vi "Select_Strings.vi"(4 "Timeout (s)":dbl=nan, 5 "Available Ch names":string[](array[string]), 6 "Message":string, 7 "Selector mode":T1(ring), 8 "Desired Ch names (in)":string[](array[string])) -> (0 "Ch Indicies Chosen":i32[](array[numeric]), 1 "Cancel":bool, 2 "Selected Channel Names":string[](array[string]))   [LabVIEW 2016]
panel:
  out "Auto-dismiss":dbl(slide) scale=0.0..60.0
  in  "Cancel 1":bool
  in  "OK":bool
  in  "Search String":string
  in  "Selector":i32[](listbox)
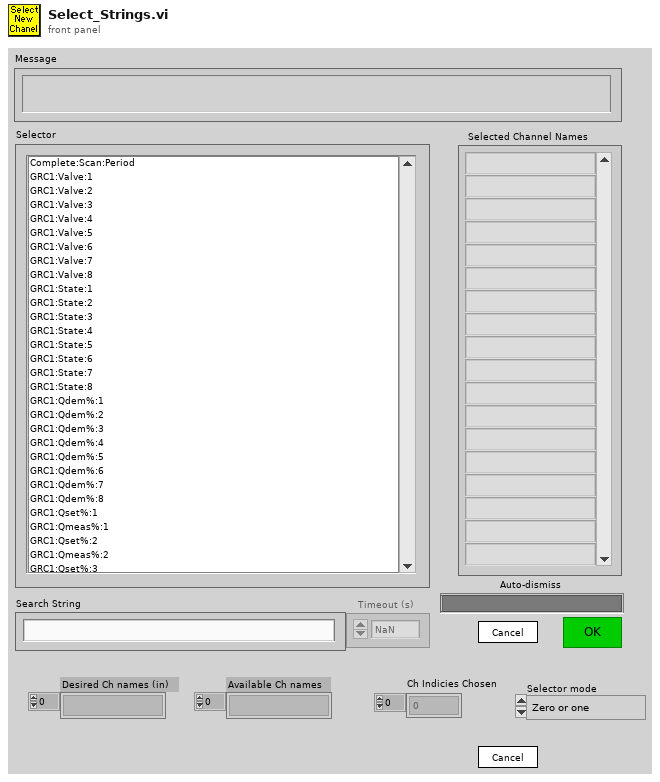
[diagram p1: front panel]
types:
  T1 = enum16{"Zero or one", "One", "Zero or more", "One or more"}
  T2 = enum8{"Enabled", "Disabled", "Disabled and Grayed Out"}
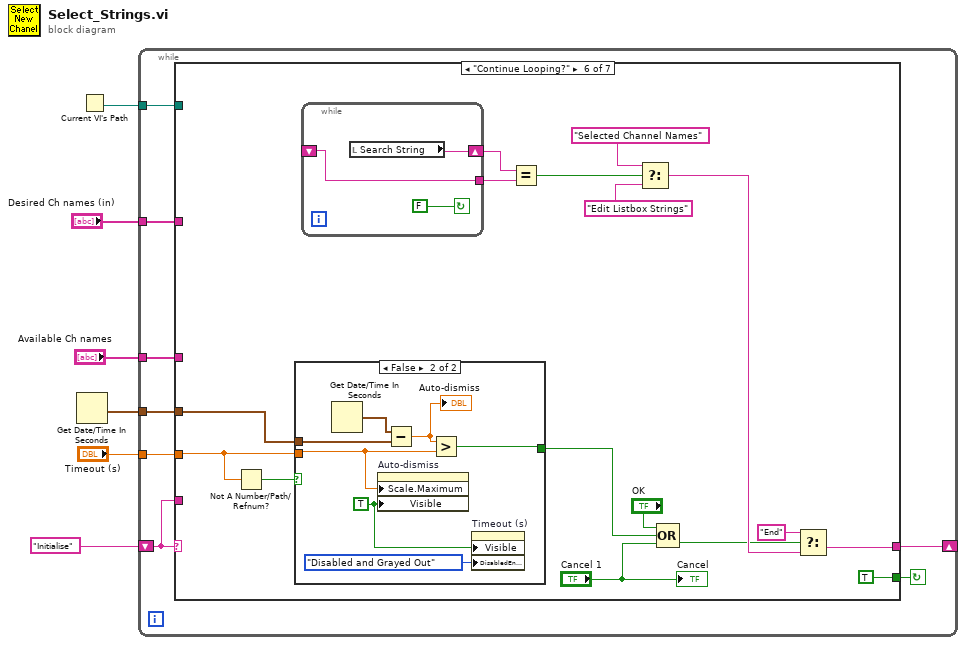
[diagram p0: block diagram]
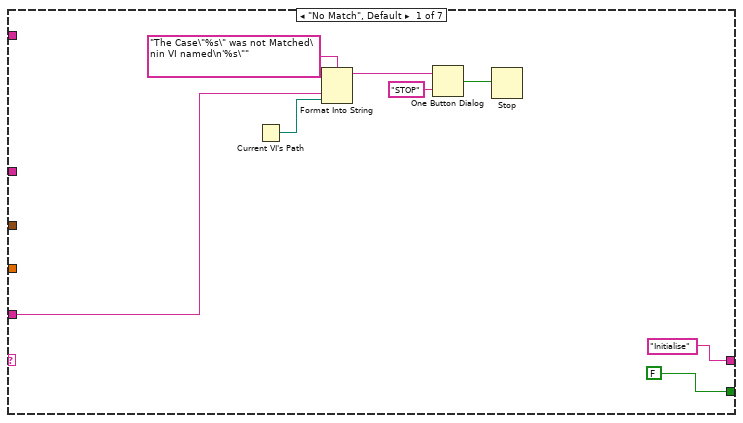
[diagram p2: hidden frame]
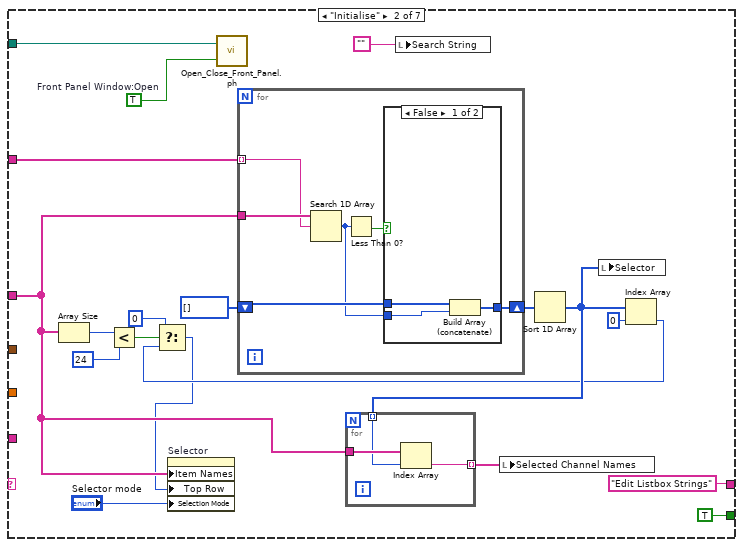
[diagram p3: hidden frame]
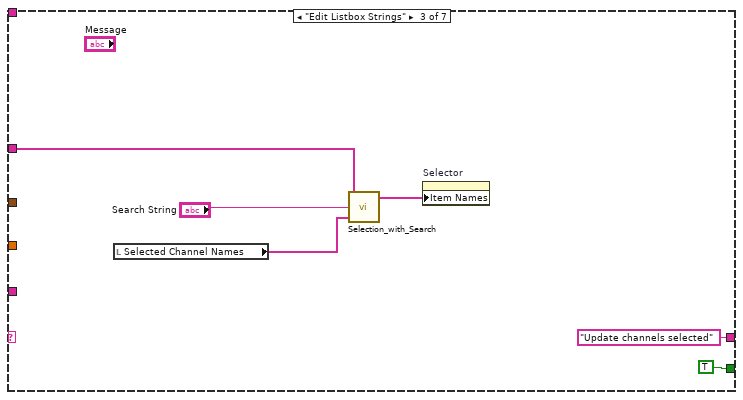
[diagram p5: hidden frame]
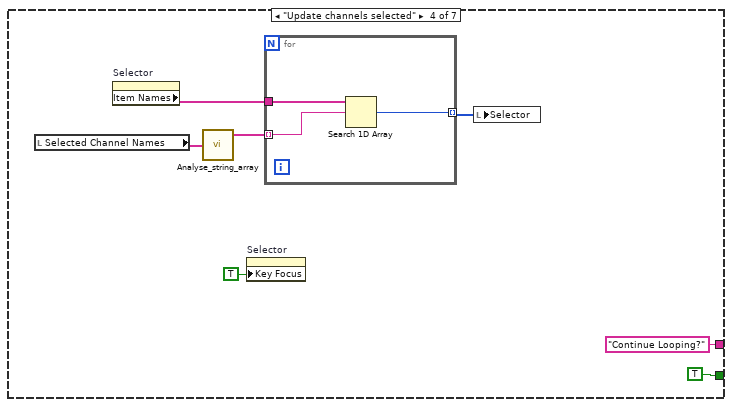
[diagram p6: hidden frame]
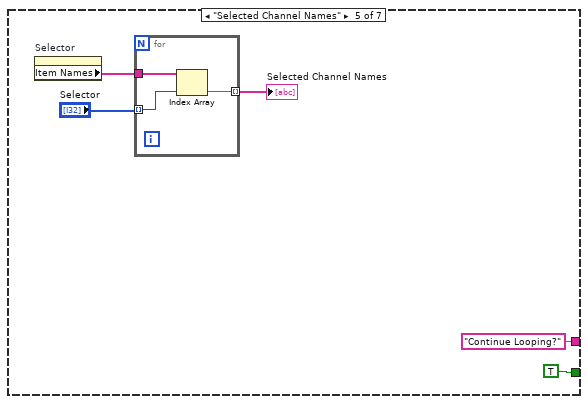
[diagram p7: hidden frame]
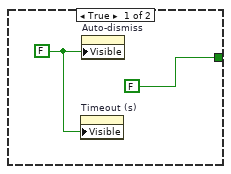
[diagram p8: hidden frame]
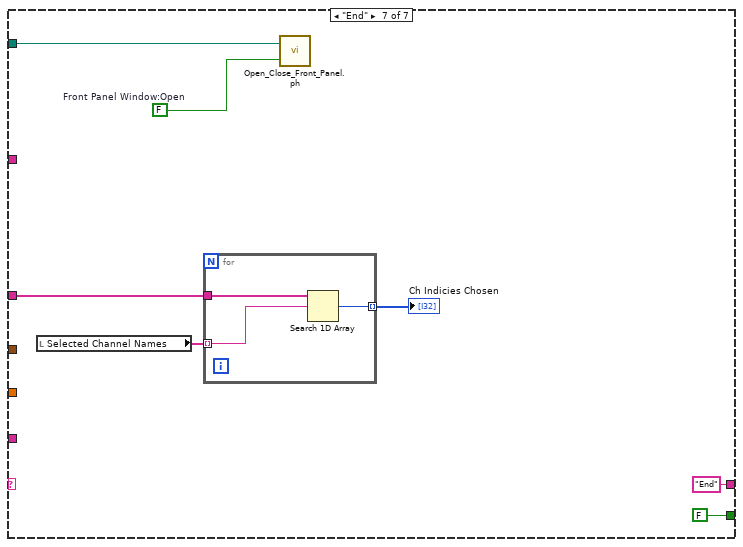
[diagram p9: hidden frame]
diagram:
  n1 = Get Date/Time In Seconds() -> (seconds since 1Jan1904=w2:timestamp)
  n2 = Current VI's Path() -> (path=w3:path)
  n3 = while {
    shift-left: "Initialise" -> [w12]
    shift-right: [w13] -> _
    tunnel: "Desired Ch names (in)" -> [w11]
    tunnel: "Available Ch names" -> [w10]
    tunnel: w3 -> [w9]
    tunnel: w2 -> [w8]
    tunnel: "Timeout (s)" -> [w7]
    stop <- w14 continue-if-true
    n4 = case shown="\"Continue Looping?\"" w12 {
      tunnel: [FALSE TRUE TRUE TRUE TRUE TRUE FALSE] -> w14
      tunnel: ["Initialise" "Edit Listbox Strings" "Update channels selected" "Continue Looping?" "Continue Looping?" w88 "End" ("t")] -> w13
      tunnel: w12 -> [w17 _ _ _ _ _ _]
      tunnel: w11 -> [_ w36 _ _ _ _ _]
      tunnel: w10 -> [_ w29 w55 _ _ _ w111]
      tunnel: w9 -> [_ w32 _ _ _ _ w108]
      tunnel: w8 -> [_ _ _ _ _ w83 _]
      tunnel: w7 -> [_ _ _ _ _ w81 _]
      frame "No Match", Default {
        n5 = Current VI's Path() -> (path=w16:path)
        n6 = Format Into String(format string="The Case\"%s\" was not Matched\nin VI named\n'%s\"" ("Format String"), w17, w16) -> (resulting string=w20:string)  [unwired: 2 in, 1 out]
        n7 = One Button Dialog(message=w20, button name ("OK")="STOP") -> (true=w18:bool)
        n8 = Stop(stop? (T)=w18) -> ()
      }
      frame "Initialise" {
        w31 = TRUE  # Front Panel Window:Open
        n9 = Array Size(array=w29) -> (size(s)=w28:i32)
        n10 = Less?(x=w28, y=24) -> (x < y?=w26:bool)
        n11 = call "Open_Close_Front_Panel.ph.vi"("Front Panel Window:Open"=w31, "VI path"=w32) -> ()  [unwired: 2 out]
        n12 = for {
          tunnel: w29 -> [w50]
          tunnel: w36 -> [w46] mode=indexing
          shift-right: [w47] -> w38
          shift-left: i32[] [] -> [w48]
          n13 = Search 1D Array(1D array=w50, element=w46) -> (index of element=w45:i32)  [unwired: 1 out]
          n14 = Less Than 0?(x=w45) -> (x < 0?=w49:bool)
          n15 = case shown="False" w49 {
            tunnel: w45 -> [w53 _]
            tunnel: w48 -> [w52 w54]
            tunnel: [w51 w54] -> w47
            frame False {
              n16 = Build Array (concatenate)(w52, w53) -> (w51:i32[])
            }
            frame True {
            }
          }
        }
        n17 = local write "Search String"("") -> ()
        n18 = Sort 1D Array(array=w38) -> (sorted array=w35:i32[])
        n19 = for {
          tunnel: w29 -> [w44]
          tunnel: w35 -> [w43] mode=indexing
          tunnel: [w42] -> w34 mode=indexing
          n20 = Index Array(array=w44, index=w43) -> (element=w42:string)
        }
        n21 = local write "Selected Channel Names"(w34) -> ()
        n22 = local write "Selector"(w35) -> ()
        n23 = Index Array(array=w35, index=0) -> (element=w25:i32)
        n24 = Select(t=0, s=w26, f=w25) -> (s? t:f=w24:i32)
        n25 = property on="Selector" class="LstBox (strict)"("Item Names"=w29, "Top Row"=w24, "Selection Mode"="Selector mode") -> ()  [unwired: 2 in, 2 out]
      }
      frame "Edit Listbox Strings" {
        n26 = local read "Selected Channel Names"() -> (w56:string[])
        n27 = call "Selection_with_Search.vi"("Selected Channel Names"=w56, "Search String"="Search String", "All Channel Names"=w55) -> ("Item Names"=w57:string[])
        n28 = property on="Selector" class="LstBox (strict)"("Item Names"=w57) -> ()  [unwired: 2 in, 2 out]
      }
      frame "Update channels selected" {
        n29 = local read "Selected Channel Names"() -> (w63:string[])
        n30 = property on="Selector" class="LstBox (strict)"() -> ("Item Names"=w65:string[])  [unwired: 2 in, 2 out]
        n31 = call "Analyse_string_array.vi"("String array"=w63) -> ("Unique strings"=w62:string[])  [unwired: 1 in, 1 out]
        n32 = property on="Selector" class="LstBox (strict)"("Key Focus"=TRUE) -> ()  [unwired: 2 in, 2 out]
        n33 = for {
          tunnel: w65 -> [w70]
          tunnel: w62 -> [w69] mode=indexing
          tunnel: [w68] -> w64 mode=indexing
          n34 = Search 1D Array(1D array=w70, element=w69) -> (index of element=w68:i32)  [unwired: 1 out]
        }
        n35 = local write "Selector"(w64) -> ()
      }
      frame "Selected Channel Names" {
        n36 = property on="Selector" class="LstBox (strict)"() -> ("Item Names"=w73:string[])  [unwired: 2 in, 2 out]
        n37 = for {
          tunnel: w73 -> [w78]
          tunnel: "Selector" -> [w77] mode=indexing
          tunnel: [w76] -> w71 mode=indexing
          n38 = Index Array(array=w78, index=w77) -> (element=w76:string)
        }
        "Selected Channel Names" <- w71
      }
      frame "Continue Looping?" {
        n39 = Not A Number/Path/Refnum?(number/path/refnum=w81) -> (NaN/Path/Refnum?=w82:bool)
        n40 = case shown="False" w82 {
          tunnel: w83 -> [_ w102]
          tunnel: w81 -> [_ w99]
          tunnel: [FALSE w101] -> w79
          frame True {
            w95 = FALSE ("Visible")
            n41 = property on="Timeout (s)" class="DigNum (strict)"("Visible"=w95) -> ()  [unwired: 2 in, 2 out]
            n42 = property on="Auto-dismiss" class="Slide (strict)"("Visible"=w95) -> ()  [unwired: 2 in, 2 out]
          }
          frame False {
            w98 = TRUE ("Visible")
            n43 = Get Date/Time In Seconds() -> (seconds since 1Jan1904=w103:timestamp)
            n44 = property on="Auto-dismiss" class="Slide (strict)"("Scale.Maximum"=w99, "Visible"=w98) -> ()  [unwired: 2 in, 2 out]
            n45 = Subtract(x=w103, y=w102) -> (x-y=w100:dbl)
            "Auto-dismiss" <- w100
            n46 = Greater?(x=w100, y=w99) -> (0:w101:bool)
            n47 = property on="Timeout (s)" class="DigNum (strict)"("Visible"=w98, "DisabledEnum"=T2."Disabled and Grayed Out" ("Disabled")) -> ()  [unwired: 2 in, 2 out]
          }
        }
        n48 = while {
          tunnel: [w105] -> w94
          shift-left: _ -> [w105]
          shift-right: [w106] -> w93
          stop <- FALSE continue-if-true
          n49 = local read "Search String"() -> (w106:string)
        }
        n50 = Equal?(x=w93, y=w94) -> (x = y?=w92:bool)
        n51 = Select(t="Selected Channel Names", s=w92, f="Edit Listbox Strings") -> (s? t:f=w87:string)
        n52 = Compound Arithmetic op=OR("OK", w79, "Cancel 1") -> (w85:bool)
        n53 = Select(t="End", s=w85, f=w87) -> (s? t:f=w88:string)
        "Cancel" <- "Cancel 1"
      }
      frame "End" {
        w107 = FALSE  # Front Panel Window:Open
        n54 = local read "Selected Channel Names"() -> (w110:string[])
        n55 = for {
          tunnel: w111 -> [w116]
          tunnel: w110 -> [w115] mode=indexing
          tunnel: [w114] -> w109 mode=indexing
          n56 = Search 1D Array(1D array=w116, element=w115) -> (index of element=w114:i32)  [unwired: 1 out]
        }
        "Ch Indicies Chosen" <- w109
        n57 = call "Open_Close_Front_Panel.ph.vi"("Front Panel Window:Open"=w107, "VI path"=w108) -> ()  [unwired: 2 out]
      }
    }
  }
